vi "Alpha4.0.3.vi"() -> ()   [LabVIEW 2011]
uses:
  <vilib>/vision/NI_Vision_Development_Module.lvlib
panel:
  in  "Operation":T1(ring)
  out "Contour":T2(plugin-control)
  in  "Look for...":u16(ring) items=["Bright Objects", "Dark Objects"]
  in  "Local Threshold Method":u16(ring) items=["Niblack", "Background Correction"]
  out "Image Enhanced":T2(plugin-control)
  in  "Gamma":sgl(slide)=2.14 scale=0.0..10.0
  in  "Contrast":u8(slide)=60 scale=0.0..255.0
  in  "Brightness":u8(slide)=118 scale=0.0..255.0
  in  "Basic Morphology Operatoin":T3(ring)=enum."Gradient in"
  out "Auto Threshold":T2(plugin-control)
  in  "Stop":bool
  in  "Browse":bool
  out "Original Image":T2(plugin-control)
  out "Path to Image":path
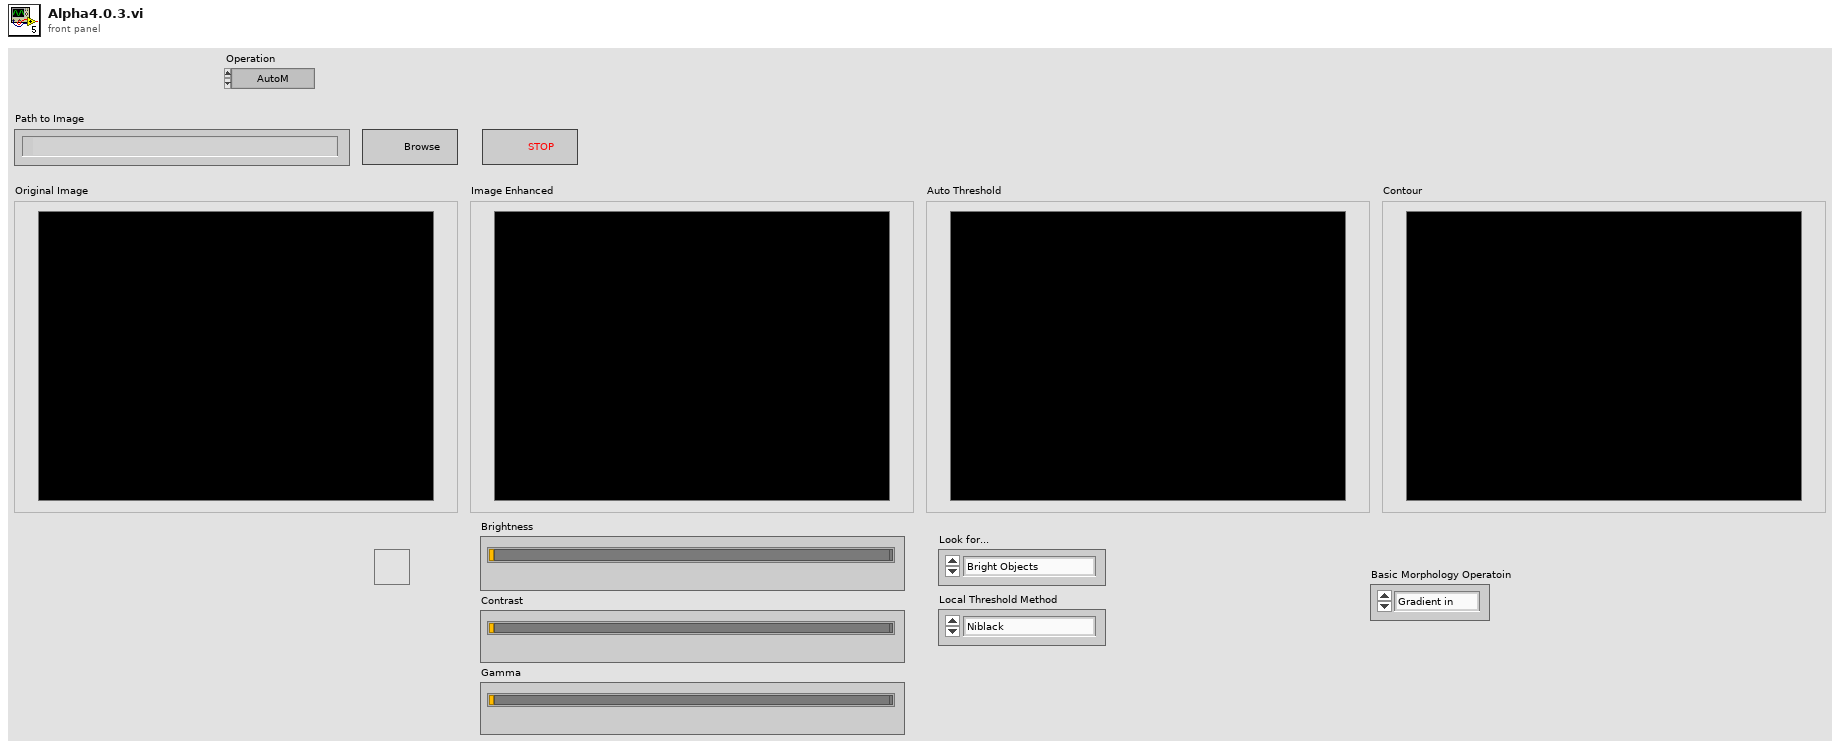
[diagram p1: front panel]
types:
  T1 = enum32{"AutoM", "Close", "Dilate", "Erode", "Gradient", "Gradient out", "Gradient in", "Hit miss", "Open", "PClose", "POpen", "Thick", "Thin"}
  T2 = typedef "IMAQ Image.ctl" = refnum<image>
  T3 = enum16{"AutoM", "Close", "Dilate", "Erode", "Gradient", "Gradient out", "Gradient in", "Hit miss", "Open", "PClose", "POpen", "Thick", "Thin"}
  T4 = typedef "Image Type" = u32
  T5 = cluster{"Brightness":u8, "Contrast":u8, "Gamma":sgl}
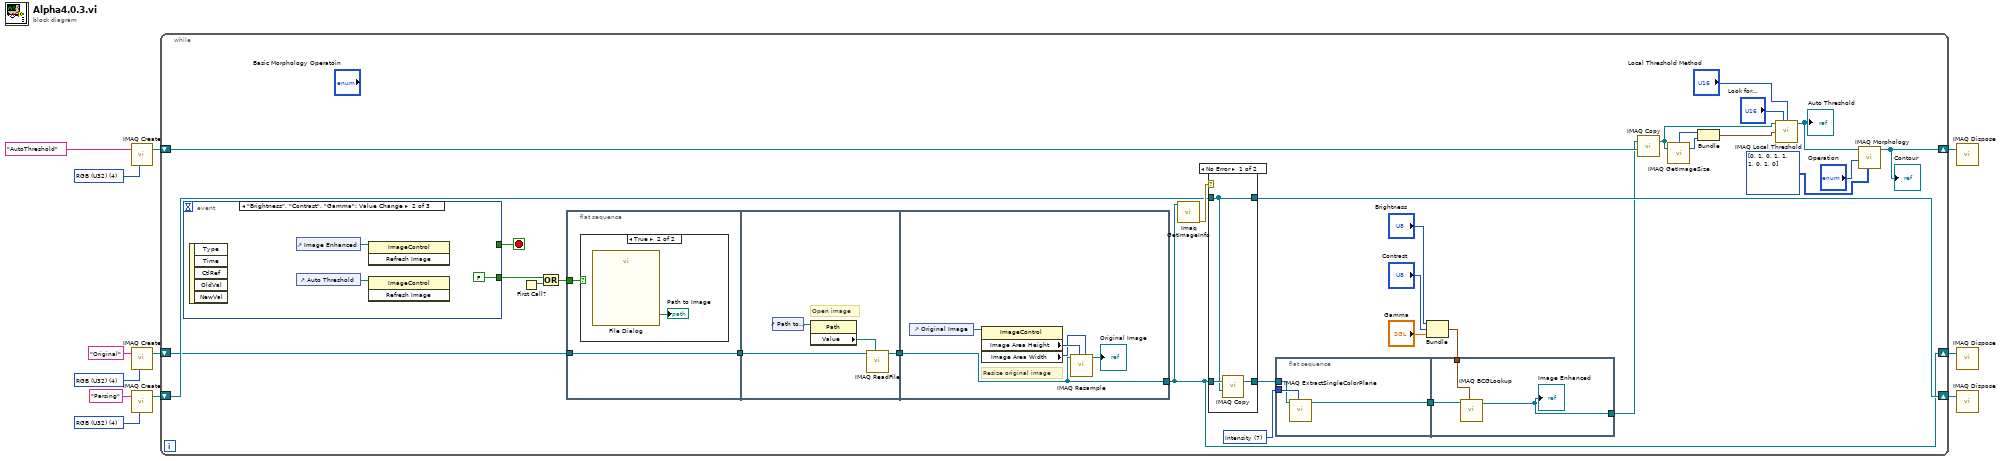
[diagram p0: block diagram]
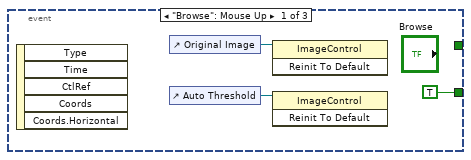
[diagram p4: hidden frame]
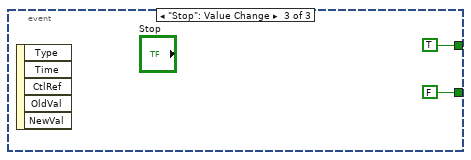
[diagram p5: hidden frame]
diagram:
  w3 = T4 4 items=["Grayscale (U8)", "Grayscale (I16)", "Grayscale (SGL)", "Complex (CSG)", "RGB (U32)", "HSL (U32)", "RGB (U64)", "Grayscale (U16)"] ("Image Type")
  w5 = T4 4 items=["Grayscale (U8)", "Grayscale (I16)", "Grayscale (SGL)", "Complex (CSG)", "RGB (U32)", "HSL (U32)", "RGB (U64)", "Grayscale (U16)"] ("Image Type")
  w8 = T4 4 items=["Grayscale (U8)", "Grayscale (I16)", "Grayscale (SGL)", "Complex (CSG)", "RGB (U32)", "HSL (U32)", "RGB (U64)", "Grayscale (U16)"] ("Image Type")
  n1 = call "IMAQ Create"("Image Name"="AutoThreshold", "Image Type"=w3) -> ("New Image"=w2:T2)  [unwired: 3 in, 1 out]
  n2 = call "IMAQ Create"("Image Name"="Original", "Image Type"=w8) -> ("New Image"=w11:T2)  [unwired: 3 in, 1 out]
  n3 = call "IMAQ Create"("Image Name"="Parsing", "Image Type"=w5) -> ("New Image"=w9:T2)  [unwired: 3 in, 1 out]
  n4 = while {
    shift-right: [w22] -> w7
    shift-left: w11 -> [w35]
    shift-right: [w28] -> w6
    shift-left: w9 -> [w39]
    shift-right: [w13] -> w1
    shift-left: w2 -> [w20]
    stop <- w40 stop-if-true
    w30 = 7 items=["Red", "Green", "Blue", "Hue", "Saturation", "Luminance", "Value", "Intensity"] ("Color Plane")
    n5 = event shown="[1] \"Brightness\", \"Contrast\", \"Gamma\": Value Change" {
      selector: _ -> [_ _ _]
      dyn-events: _ -> [_ _ _]
      timeout: _ -> [_ _ _]
      tunnel: [_ _ TRUE] -> w40
      tunnel: [TRUE FALSE FALSE] -> w38
      event "Browse": Mouse Up {
        n6 = event-data() -> ()  [unwired: 1 in, 5 out]
        n7 = control-ref of="Original Image"() -> (w67:refnum<vi>)
        n8 = control-ref of="Auto Threshold"() -> (w68:refnum<vi>)
        n9 = invoke class="ImageControl" method="Reinit To Default"(reference=w67) -> ()  [unwired: 2 in, 3 out]
        n10 = invoke class="ImageControl" method="Reinit To Default"(reference=w68) -> ()  [unwired: 2 in, 3 out]
      }
      event "Brightness", "Contrast", "Gamma": Value Change {
        n11 = event-data() -> ()  [unwired: 1 in, 5 out]
        n12 = control-ref of="Image Enhanced"() -> (w71:refnum<vi>)
        n13 = control-ref of="Auto Threshold"() -> (w69:refnum<vi>)
        n14 = invoke class="ImageControl" method="Refresh Image"(reference=w71) -> ()  [unwired: 2 in, 3 out]
        n15 = invoke class="ImageControl" method="Refresh Image"(reference=w69) -> ()  [unwired: 2 in, 3 out]
      }
      event "Stop": Value Change {
        n16 = event-data() -> ()  [unwired: 1 in, 5 out]
      }
    }
    n17 = First Call?() -> (First Call?: T/F=w37:bool)
    n18 = Or(x=w38, y=w37) -> (x .or. y?=w36:bool)
    n19 = flat-sequence {
      tunnel: w36 -> [w55]
      tunnel: w35 -> [w54]
      tunnel: [w54] -> w34
      tunnel: [w60] -> w42
      tunnel: w34 -> [w57]
      tunnel: w42 -> [w61]
      tunnel: [w61] -> w22
      frame #0 {
        n20 = case shown="True" w55 {
          frame False {
          }
          frame True {
            n21 = call "File Dialog"() -> ("selected path"=→"Path to Image":path)  [unwired: 12 in, 3 out]
          }
        }
      }
      frame #1 {
        # "Open image"
        n22 = control-ref of="Path to Image"() -> (w59:refnum<vi>)
        n23 = property class="Path"(reference=w59) -> ("Value"=w58:path)  [unwired: 1 in, 2 out]
        n24 = call "IMAQ ReadFile"("File Path"=w58, "Image"=w57) -> ("Image Out"=w60:T2)  [unwired: 5 in, 4 out]
      }
      frame #2 {
        # "Resize original image"
        n25 = control-ref of="Original Image"() -> (w65:refnum<vi>)
        n26 = property class="ImageControl"(reference=w65) -> ("Image Area Height"=w64:u32, "Image Area Width"=w63:u32)  [unwired: 1 in, 2 out]
        n27 = call "IMAQ Resample"("X Resolution"=w63, "Y Resolution"=w64, "Image Src"=w61) -> ("Image Dst Out"=→"Original Image":T2)  [unwired: 7 in, 1 out]
      }
    }
    n28 = call "Imaq GetImageInfo"("Image"=w22) -> ("error out"=w41:errorcluster)  [unwired: 1 in, 9 out]
    n29 = case shown="No Error" w41 {
      tunnel: w39 -> [w49 w52]
      tunnel: w22 -> [w51 w53]
      tunnel: [w50 w53] -> w29
      tunnel: [w49 w52] -> w28
      frame No Error {
        n30 = call "IMAQ Copy"("Image Dst"=w49, "Image Src"=w51) -> ("Image Dst Out"=w50:T2)  [unwired: 4 in, 1 out]
      }
      frame Error {
      }
    }
    n31 = flat-sequence {
      tunnel: w30 -> [w44]
      tunnel: w29 -> [w43]
      tunnel: [w45] -> w19
      tunnel: [w47] -> w17
      tunnel: w19 -> [w46]
      tunnel: w18 -> [w48]
      frame #0 {
        n32 = call "IMAQ ExtractSingleColorPlane"("Color Plane"=w44, "Image Src"=w43) -> ("Image Dst Out"=w45:T2)  [unwired: 2 in, 7 out]
      }
      frame #1 {
        n33 = call "IMAQ BCGLookup"("Image Src"=w46, "BCG Values"=w48) -> ("Image Dst Out"=w47:T2)  [unwired: 3 in, 3 out]
        "Image Enhanced" <- w47
      }
    }
    n34 = Bundle("Brightness"="Brightness", "Contrast"="Contrast", "Gamma"="Gamma") -> (w18:T5)  [unwired: 1 in]
    n35 = call "IMAQ Copy"("Image Dst"=w20, "Image Src"=w17) -> ("Image Dst Out"=w21:T2)  [unwired: 4 in, 1 out]
    n36 = call "IMAQ GetImageSize"("Image"=w21) -> ("Y Resolution"=w24:i32, "X Resolution"=w25:i32)  [unwired: 1 in, 3 out]
    n37 = Bundle("X Resolution"=w25, "Y Resolution"=w24) -> (w26:cluster{"X Resolution":i32, "Y Resolution":i32})  [unwired: 1 out]
    n38 = call "IMAQ Local Threshold"("Image Src"=w21, "Look For (Bright Objects)"="Look for...", "Method (Niblack)"="Local Threshold Method", "Window Size (32x32)"=w26) -> ("Image Dst Out"=w16:T2)  [unwired: 10 in, 1 out]
    "Auto Threshold" <- w16
    n39 = call "IMAQ Morphology"("Structuring Element"=i32[][] [[0, 1, 0], [1, 1, 1], [0, 1, 0]], "Operation"="Operation", "Image Src"=w16) -> ("Image Dst Out"=w13:T2)  [unwired: 7 in, 1 out]
    "Contour" <- w13
  }
  n40 = call "IMAQ Dispose"("Image"=w1) -> ()  [unwired: 5 in, 1 out]
  n41 = call "IMAQ Dispose"("Image"=w7) -> ()  [unwired: 5 in, 1 out]
  n42 = call "IMAQ Dispose"("Image"=w6) -> ()  [unwired: 5 in, 1 out]
